vi "Get and Intitialize CPID Channel References.vi"(8 "error in (no error)":errorcluster, 10 "Refs":T4[](array[typedef]) {"Signal Refs" format="%.0x"}, 11 "Item Ref in":T3 format="%.0x") -> (0 "error out":errorcluster, 1 "output cluster":cluster{"Refs":T1[], "Values":dbl[]} {"Refs"."Data Reference" format="%.0x"}, 2 "Lookup Table":variant, 3 "Item Ref out":T3=18446744073709551615 format="%.0x")   [LabVIEW 2015, in "Diagnostics Addon Engine.lvlib"]
uses:
  Diagnostics Addon Engine.lvlib
  <vilib>/NI Veristand/Custom Device API/Custom Device Item Ref.ctl
  DIDPID Signal VS References.ctl
  <vilib>/NI Veristand/Custom Device API/Block Data Reference.ctl
  <vilib>/NI Veristand/Custom Device API/Data Reference.ctl
  <vilib>/NI Veristand/Custom Device API/Data Access Type.ctl
  Datatable Lookup Positions.ctl
  <vilib>/NI Veristand/Custom Device API/Custom Device API.lvlib
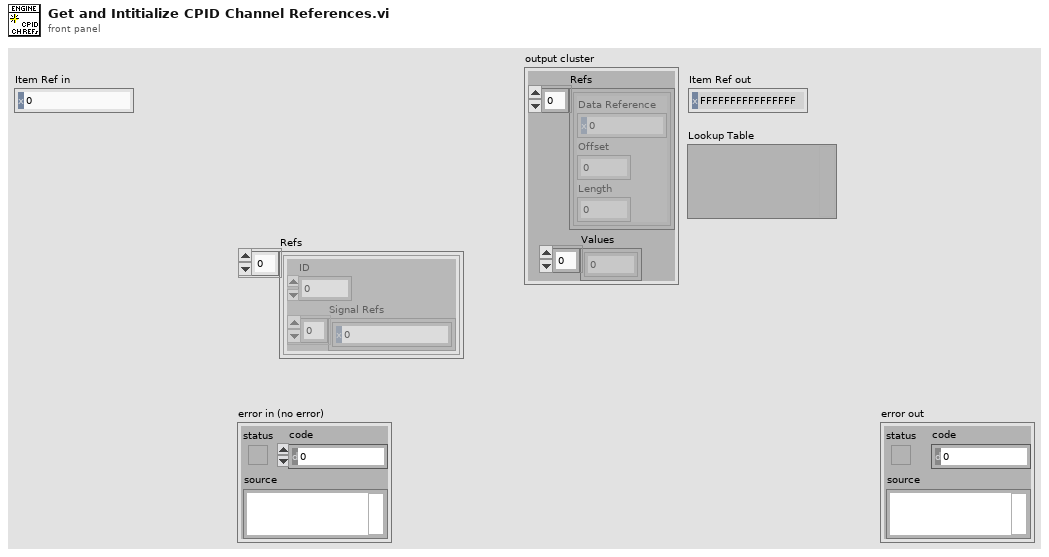
[diagram p1: front panel]
types:
  T1 = typedef "Custom Device API.lvlib/Block Data Reference.ctl" = cluster{"Data Reference":T2, "Offset":u64, "Length":u64}
  T2 = typedef "Custom Device API.lvlib/Data Reference.ctl" = i32
  T3 = typedef "Custom Device API.lvlib/Custom Device Item Ref.ctl" = u64
  T4 = typedef "Diagnostics Addon Engine.lvlib/DIDPID Signal VS References.ctl" = cluster{"ID":u16, "Signal Refs":T3[]}
  T5 = typedef "Custom Device API.lvlib/Data Access Type.ctl" = enum16{"Read", "Write"}
  T6 = typedef "Diagnostics Addon Engine.lvlib/Datatable Lookup Positions.ctl" = cluster{"Offset":i32, "Length":i32}
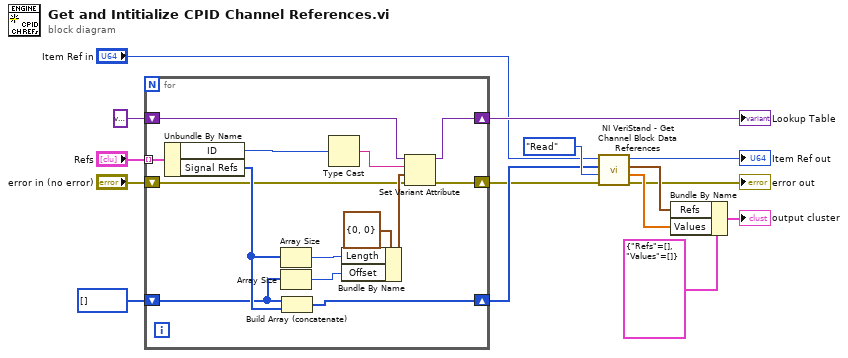
[diagram p0: block diagram]
diagram:
  n1 = for {
    tunnel: "Refs" -> [w21] mode=indexing
    shift-right: [w22] -> w12
    shift-left: variant -> [w26]
    shift-right: [w24] -> w4
    shift-left: "error in (no error)" -> [w16]
    shift-right: [w19] -> w9
    shift-left: T3[] [] -> [w17]
    n2 = Unbundle By Name(w21) -> ("ID"=w20:u16, "Signal Refs"=w18:T3[])
    n3 = Array Size(array=w18) -> (size(s)=w29:i32)
    n4 = Array Size(array=w17) -> (size(s)=w25:i32)
    n5 = Build Array (concatenate)(w17, w18) -> (w19:T3[])
    n6 = Type Cast(x=w20) -> (*(type *) &x=w23:string)  [unwired: 1 in]
    n7 = Bundle By Name(cluster=T6 {"Offset"=0, "Length"=0}, "Length"=w29, "Offset"=w25) -> (w27:T6)
    n8 = Set Variant Attribute(Variant=w26, name=w23, value=w27, error in=w16) -> (Variant out=w22:variant, error out=w24:errorcluster)  [unwired: 1 out]
  }
  "Lookup Table" <- w12
  n9 = call <vilib>:"NI VeriStand - Get Channel Block Data References.vi"("error in (no error)"=w4, "Access"=Data_Access_Type."Read", "Channel Refs"=w9, "Device Ref in"="Item Ref in") -> ("error out"=→"error out":errorcluster, "Values Array"=w5:dbl[], "Block Data Refs"=w6:T1[], "Device Ref out"=→"Item Ref out":T3)  [unwired: 4 in]
  n10 = Bundle By Name(cluster=cluster{"Refs":T1[], "Values":dbl[]} {"Refs"=[], "Values"=[]} ("Pairs"), "Refs"=w6, "Values"=w5) -> (→"output cluster":cluster{"Refs":T1[], "Values":dbl[]})
